vi "Set AIM Hardware Parameters.vi"(8 "error in":errorcluster, 10 "aim hardware parameters":T1={"initialization method"=enum."PXI Slot Number", "card number"=0, "pxi slot number"=2, "biu number"=0, "bus selection"=enum."Both", "coupling mode"=enum."Isolated Onboard Termination"}, 11 "custom device":T5=18446744073709551615 format="%.0x") -> (0 "error out":errorcluster, 3 "custom device out":T5 format="%.0x")   [LabVIEW 2020, in "AIM MIL-STD-1553 Scripting.lvlib"]
doc: "Configures <b>aim hardware parameters</b> such as PXI Slot Number and BIU Number in the system definition for the specified <b>custom device</b>."
uses:
  AIM MIL-STD-1553 Scripting.lvlib
  <vilib>/NI VeriStand/Custom Device API/Custom Device Item Ref.ctl
  Shared/AIM Hardware Parameters.ctl
  Shared/Initialization Method.ctl
  Shared/Bus Selection.ctl
  Shared/Coupling Mode.ctl
  Constants.vi
  <vilib>/NI VeriStand/Custom Device API/Set Item Property (U16).vi
  <vilib>/NI VeriStand/Custom Device API/Set Item Property (I32).vi
  <vilib>/NI VeriStand/Custom Device API/Custom Device API.lvlib
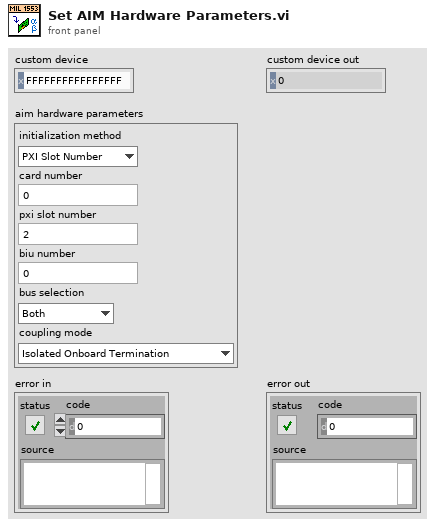
[diagram p1: front panel]
types:
  T1 = typedef "AIM Hardware Parameters.ctl" = cluster{"initialization method":T2, "card number":i32, "pxi slot number":i32, "biu number":i32, "bus selection":T3, "coupling mode":T4}
  T2 = typedef "Initialization Method.ctl" = enum16{"PXI Slot Number", "Card Number"}
  T3 = typedef "Bus Selection.ctl" = enum16{"Both", "Primary", "Secondary"}
  T4 = typedef "Coupling Mode.ctl" = enum16{"Isolated Onboard Termination", "Transformer Coupled", "Direct Coupled", "External with Onboard Termination", "Onboard Digital Wrap-around"}
  T5 = typedef "Custom Device API.lvlib/Custom Device Item Ref.ctl" = u64
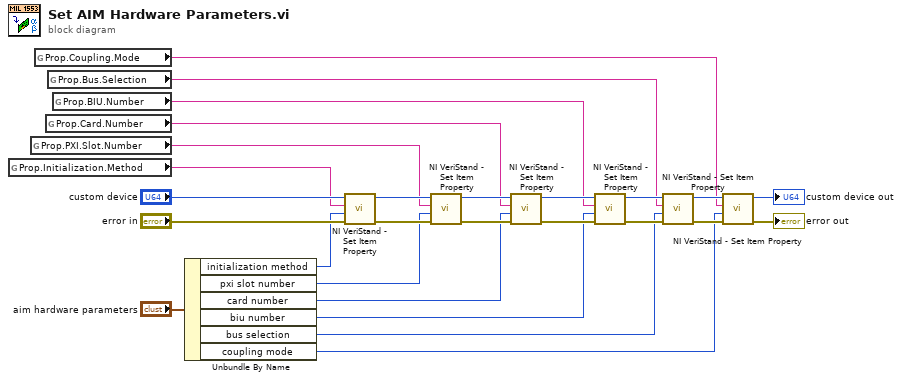
[diagram p0: block diagram]
diagram:
  n1 = global read "Constants.vi" "Prop.Initialization.Method"() -> (w15:string)
  n2 = global read "Constants.vi" "Prop.PXI.Slot.Number"() -> (w14:string)
  n3 = global read "Constants.vi" "Prop.Coupling.Mode"() -> (w3:string)
  n4 = global read "Constants.vi" "Prop.Card.Number"() -> (w13:string)
  n5 = global read "Constants.vi" "Prop.Bus.Selection"() -> (w4:string)
  n6 = global read "Constants.vi" "Prop.BIU.Number"() -> (w12:string)
  n7 = Unbundle By Name("aim hardware parameters") -> ("initialization method"=w19:T2, "pxi slot number"=w18:i32, "card number"=w17:i32, "biu number"=w16:i32, "bus selection"=w1:T3, "coupling mode"=w2:T4)
  n8 = call-poly <vilib>:"NI VeriStand - Set Item Property.vi"("error in (no error)"="error in", "Value"=w19, "Property Name"=w15, "Item Ref in"="custom device") -> ("error out"=w21:errorcluster, "Item Ref out"=w20:T5)  [unwired: 5 in, 1 out]
  n9 = call-poly <vilib>:"NI VeriStand - Set Item Property.vi"("error in (no error)"=w21, "Value"=w18, "Property Name"=w14, "Item Ref in"=w20) -> ("error out"=w26:errorcluster, "Item Ref out"=w27:T5)  [unwired: 5 in, 1 out]
  n10 = call-poly <vilib>:"NI VeriStand - Set Item Property.vi"("error in (no error)"=w26, "Value"=w17, "Property Name"=w13, "Item Ref in"=w27) -> ("error out"=w24:errorcluster, "Item Ref out"=w25:T5)  [unwired: 5 in, 1 out]
  n11 = call-poly <vilib>:"NI VeriStand - Set Item Property.vi"("error in (no error)"=w24, "Value"=w16, "Property Name"=w12, "Item Ref in"=w25) -> ("error out"=w8:errorcluster, "Item Ref out"=w5:T5)  [unwired: 5 in, 1 out]
  n12 = call-poly <vilib>:"NI VeriStand - Set Item Property.vi"("error in (no error)"=w8, "Value"=w1, "Property Name"=w4, "Item Ref in"=w5) -> ("error out"=w10:errorcluster, "Item Ref out"=w9:T5)  [unwired: 5 in, 1 out]
  n13 = call-poly <vilib>:"NI VeriStand - Set Item Property.vi"("error in (no error)"=w10, "Value"=w2, "Property Name"=w3, "Item Ref in"=w9) -> ("error out"=→"error out":errorcluster, "Item Ref out"=→"custom device out":T5)  [unwired: 5 in, 1 out]
